vi "Autonomous State Machine.vi"   [LabVIEW 2014]
doc: "This VI is called when autonomous begins, and will automatically be terminated when autonomous ends. You can carry out timed or sensor driven robot movement independently without needing to return to the caller."
panel:
  # "Be sure to right-click and choose Data Operations>>Make Current Value default if you want to save the array values with the VI"
types:
  T1 = typedef "WPI_MotorControlDeviceRef.ctl" = cluster{"DeviceStatus":errorcluster, "Type":T2, "PWM":cluster{"Controller":T3, "PWM Channel":T4, "DeadBand":T5}, "CAN":cluster{"Device Number":u8, "Control Mode":T6, "Semaphore":T7, "Max Vout":dbl, "TalonSRX Control Mode":T8}, "Invert":bool, "TransformRef":T9, "InvTransformRef":T9}
  T2 = typedef "WPI_MotorControlType.ctl" = enum16{"PWM", "CAN", "CANTalonSRX"}
  T3 = typedef "FPGA_TypedefDigitalModule.ctl" = enum16{"Controller 1"}
  T4 = typedef "FPGA_DIOPWMChannel.ctl" = enum8{"PWM 0", "PWM 1", "PWM 2", "PWM 3", "PWM 4", "PWM 5", "PWM 6", "PWM 7", "PWM 8", "PWM 9", "PWM MXP 0", "PWM MXP 1", "PWM MXP 2", "PWM MXP 3", "PWM MXP 4", "PWM MXP 5", "PWM MXP 6", "PWM MXP 7", "PWM MXP 8", "PWM MXP 9", "Invalid"}
  T5 = typedef "WPI_PWMDeadband.ctl" = cluster{"Name":string, "maxPositivePwm":i32, "minPositivePwm":i32, "centerPwm":i32, "maxNegativePwm":i32, "minNegativePwm":i32, "angularRange":u16}
  T6 = typedef "WPI_CANJaguar_ControlMode.ctl" = enum8{"Percent VBus", "Current", "Speed", "Position", "Voltage"}
  T7 = typedef "Semaphore RefNum" = refnum<k1>
  T8 = typedef "WPI_CANTalonSRX_APIControlMode.ctl" = enum8{"Percent VBus", "Speed", "Position", "Slave", "Unchanged / Invalid"}
  T9 = typedef "WPI_PWMTransform_ConPane.ctl" = refnum<vi>
  T10 = typedef "WPI_DigitalInputDevRef.ctl" = cluster{"DevStatus":errorcluster, "DIO Channel":T11, "Controller":T3}
  T11 = typedef "FPGA_DIOChannel.ctl" = enum8{"DIO 0", "DIO 1", "DIO 2", "DIO 3", "DIO 4", "DIO 5", "DIO 6", "DIO 7", "DIO 8", "DIO 9", "DIO MXP 0", "DIO MXP 1", "DIO MXP 2", "DIO MXP 3", "DIO MXP 4", "DIO MXP 5", "DIO MXP 6", "DIO MXP 7", "DIO MXP 8", "DIO MXP 9", "DIO MXP 10", "DIO MXP 11", "DIO MXP 12", "DIO MXP 13", "DIO MXP 14", "DIO MXP 15", "Invalid"}
  T12 = typedef "WPI_RobotDriveDevRef.ctl" = cluster{"DevStatus":errorcluster, "Motors[]":T1[], "Square Inputs":bool, "Max Output":dbl}
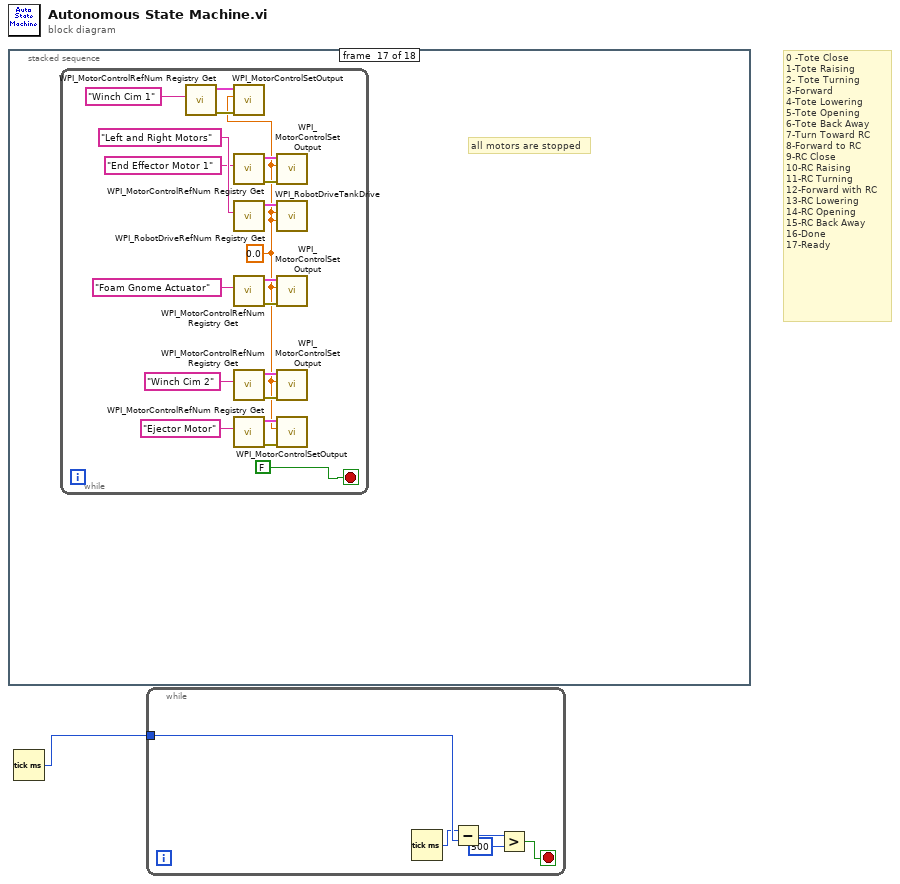
[diagram p0: block diagram]
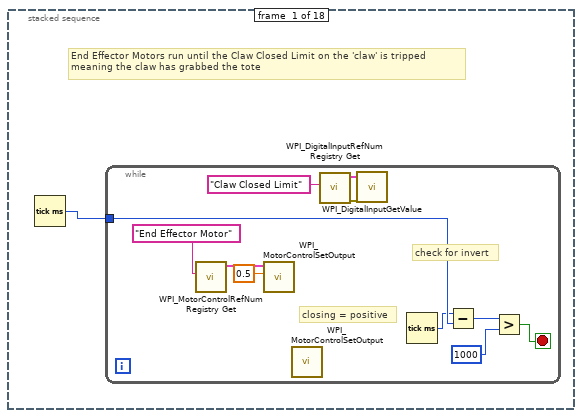
[diagram p2: hidden frame]
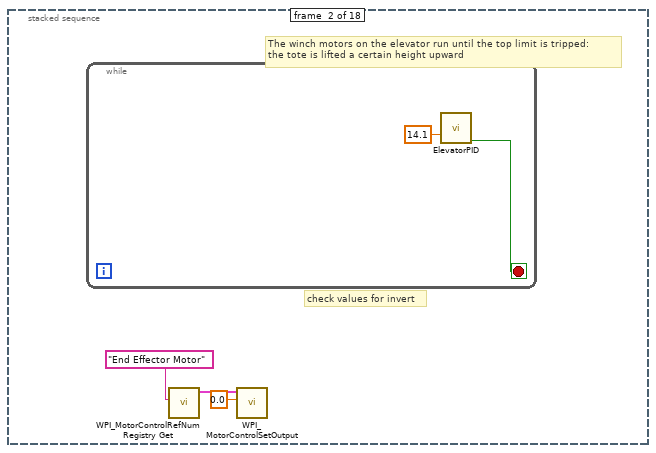
[diagram p3: hidden frame]
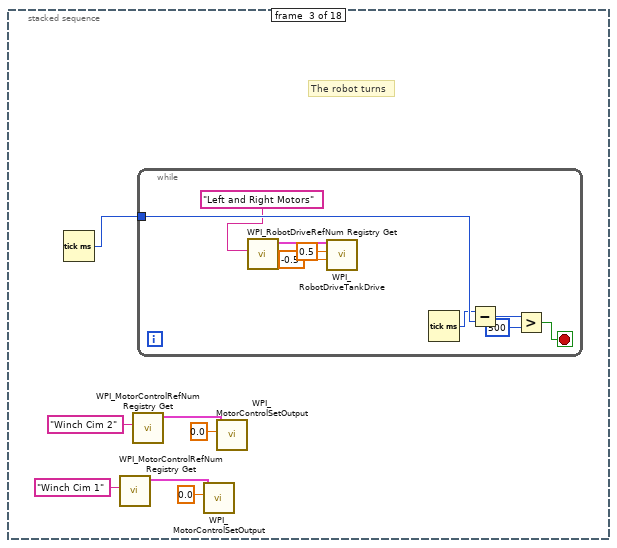
[diagram p4: hidden frame]
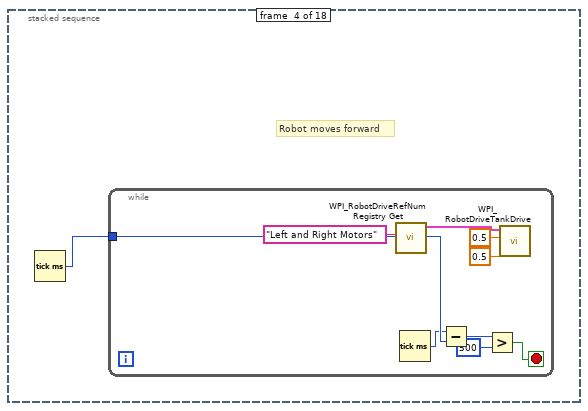
[diagram p5: hidden frame]
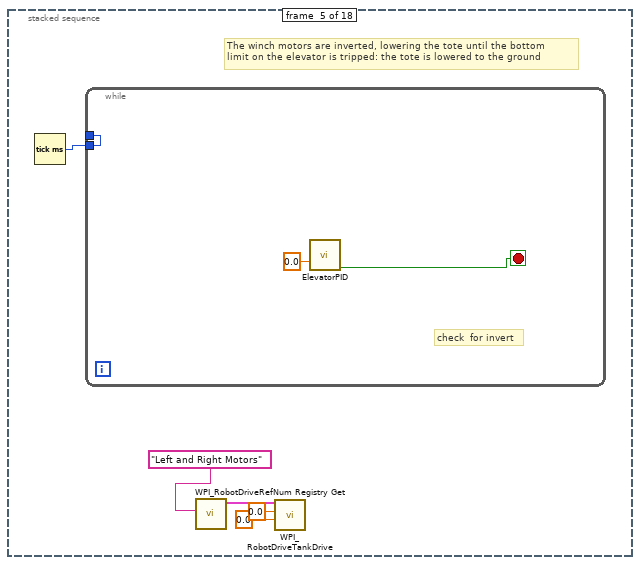
[diagram p6: hidden frame]
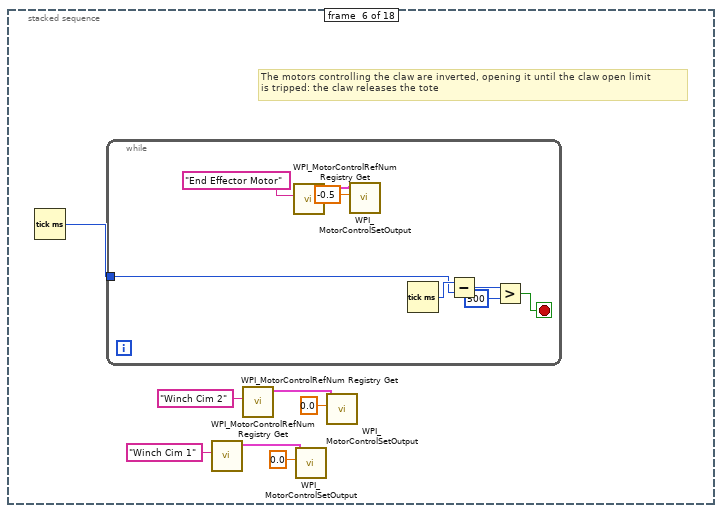
[diagram p7: hidden frame]
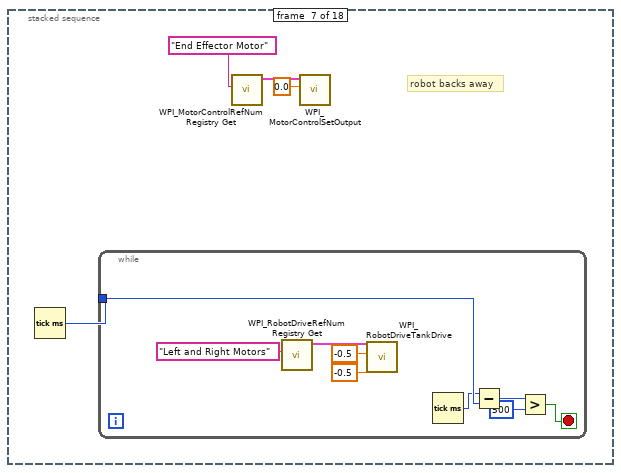
[diagram p8: hidden frame]
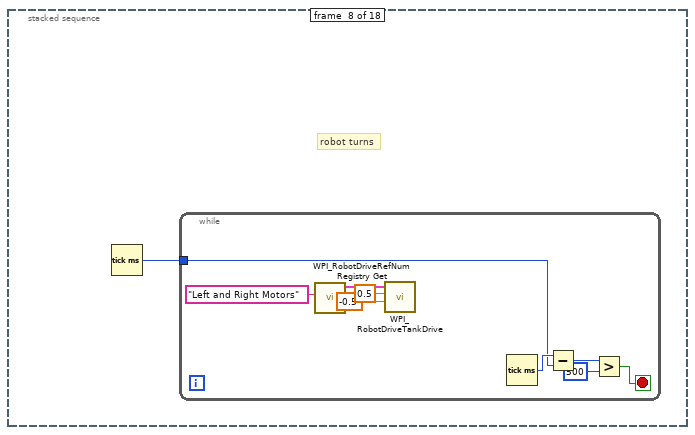
[diagram p9: hidden frame]
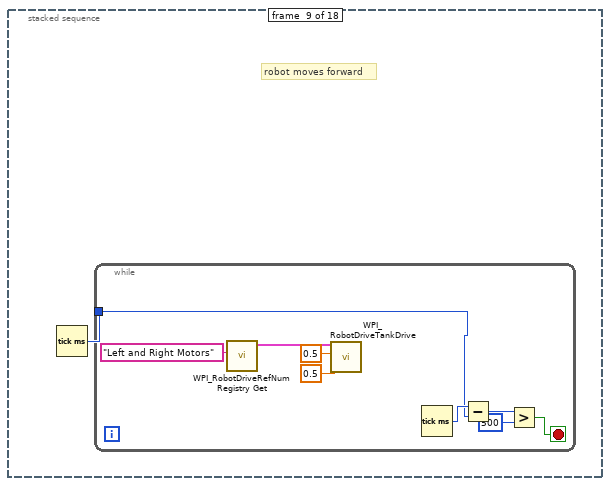
[diagram p10: hidden frame]
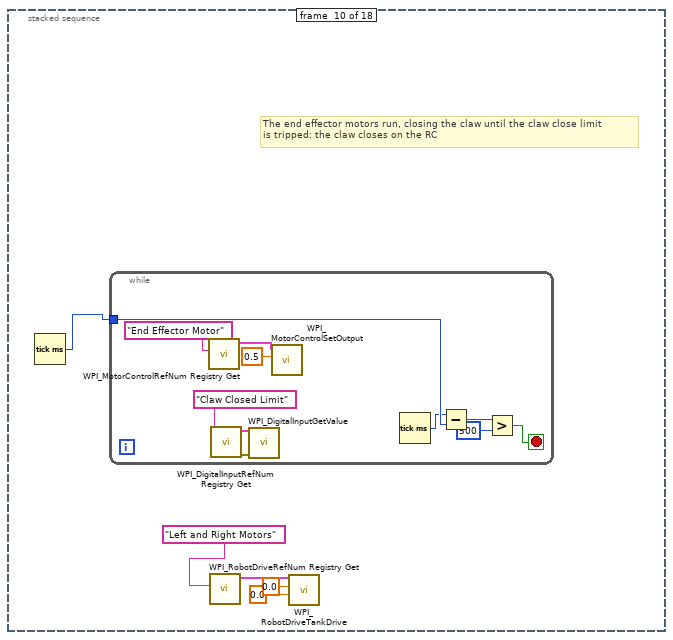
[diagram p11: hidden frame]
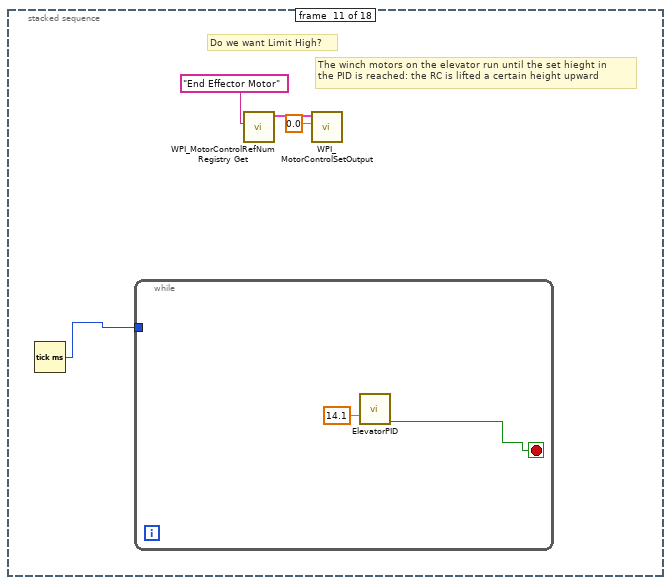
[diagram p12: hidden frame]
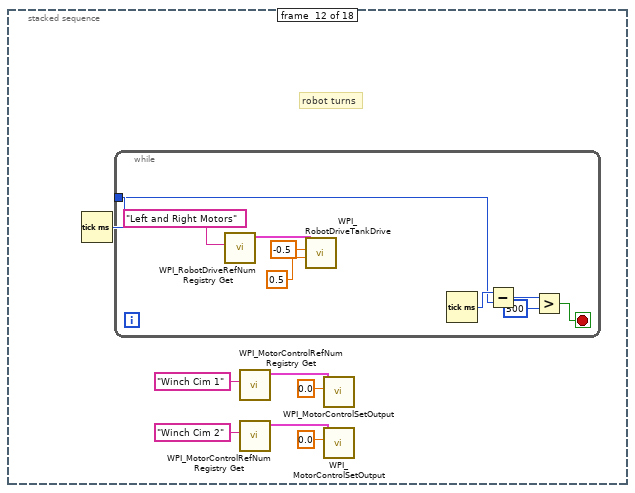
[diagram p13: hidden frame]
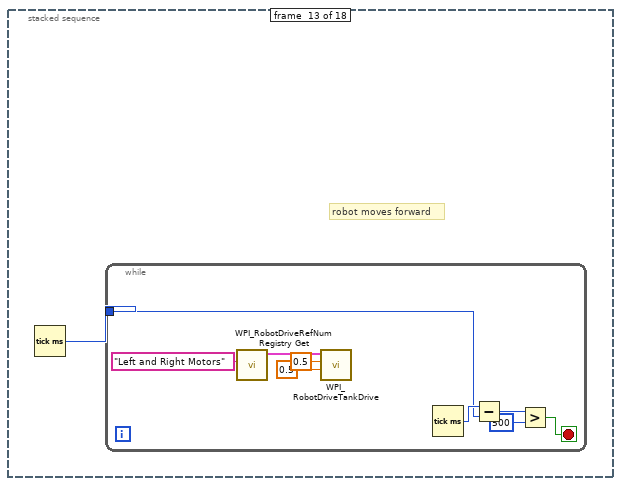
[diagram p14: hidden frame]
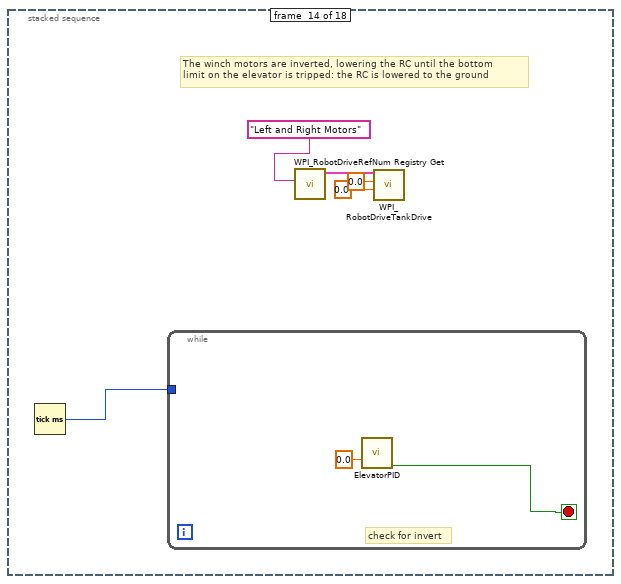
[diagram p15: hidden frame]
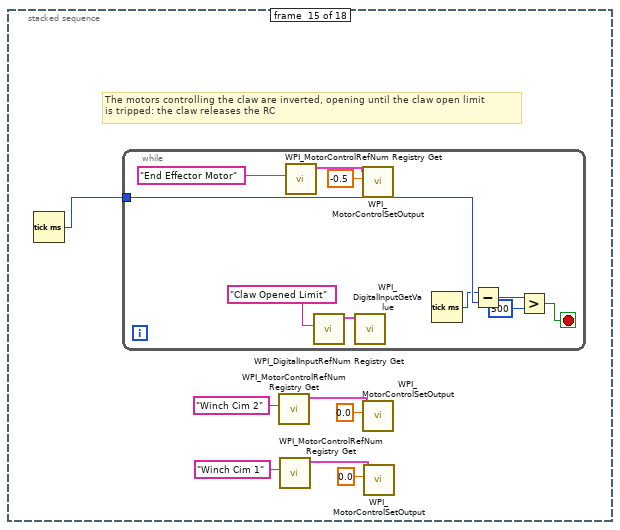
[diagram p16: hidden frame]
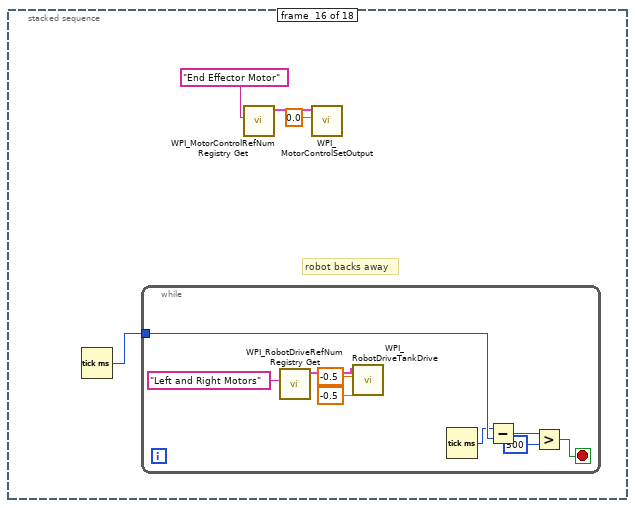
[diagram p17: hidden frame]
diagram:
  # "0 -Tote Close\n1-Tote Raising\n2- Tote Turning\n3-Forward\n4-Tote Lowering\n5-Tote Opening\n6-Tote Back Away\n7-Turn Toward RC\n8-Forward to RC\n9-RC Close\n10-RC Raising\n11-RC Turning\n12-Forward with RC\n13-RC Lowering\n14-RC Opening\n15-RC Back Away\n16-Done\n17-Ready"
  n1 = stacked-sequence {
    frame #0 {
      # "End Effector Motors run until the Claw Closed Limit on the 'claw' is tripped\nmeaning the claw has grabbed the tote"
      n2 = Tick Count (ms)() -> (millisecond timer value=w2:u32)
      n3 = while {
        tunnel: w2 -> [w10]
        stop <- w11 stop-if-true
        # "closing = positive"
        # "check for invert"
        n4 = call <vilib>:"WPI_MotorControlRefNum Registry Get.vi"("refnum name"="End Effector Motor") -> ("MotorControlDevRef"=w6:T1)  [unwired: 9 in, 1 out]
        n5 = call <vilib>:"WPI_MotorControlSetOutput.vi"("Output"=0.5, "MotorControlDevRef"=w6) -> ()  [unwired: 7 in, 3 out]
        n6 = call <vilib>:"WPI_MotorControlSetOutput.vi"() -> ()  [unwired: 9 in, 3 out]
        n7 = call <vilib>:"WPI_DigitalInputRefNum Registry Get.vi"("refnum name"="Claw Closed Limit") -> ("error out"=w4:errorcluster, "DigitalInputDevRef"=w3:T10)  [unwired: 9 in]
        n8 = call <vilib>:"WPI_DigitalInputGetValue.vi"("error in (no error)"=w4, "DigitalInputDevRef"=w3) -> ()  [unwired: 7 in, 3 out]
        n9 = Tick Count (ms)() -> (millisecond timer value=w9:u32)
        n10 = Subtract(x=w9, y=w10) -> (x-y=w13:u32)
        n11 = Greater?(x=w13, y=u32 1000) -> (0:w11:bool)
      }
    }
    frame #1 {
      # "The winch motors on the elevator run until the top limit is tripped: \nthe tote is lifted a certain height upward"
      # "check values for invert"
      n12 = while {
        stop <- w18 stop-if-true
        n13 = call "ElevatorPID.vi"("Elevator Setpoint"=14.1) -> ("At Setpoint"=w18:bool)  [unwired: 14 in]
      }
      n14 = call <vilib>:"WPI_MotorControlRefNum Registry Get.vi"("refnum name"="End Effector Motor") -> ("MotorControlDevRef"=w14:T1)  [unwired: 9 in, 1 out]
      n15 = call <vilib>:"WPI_MotorControlSetOutput.vi"("Output"=0.0, "MotorControlDevRef"=w14) -> ()  [unwired: 7 in, 3 out]
    }
    frame #2 {
      # "The robot turns"
      n16 = Tick Count (ms)() -> (millisecond timer value=w25:u32)
      n17 = call <vilib>:"WPI_MotorControlRefNum Registry Get.vi"("refnum name"="Winch Cim 1") -> ("MotorControlDevRef"=w20:T1)  [unwired: 9 in, 1 out]
      n18 = call <vilib>:"WPI_MotorControlRefNum Registry Get.vi"("refnum name"="Winch Cim 2") -> ("MotorControlDevRef"=w23:T1)  [unwired: 9 in, 1 out]
      n19 = while {
        tunnel: w25 -> [w31]
        stop <- w32 stop-if-true
        n20 = call <vilib>:"WPI_RobotDriveRefNum Registry Get.vi"("refnum name"="Left and Right Motors") -> ("RobotDriveDevRef"=w29:T12)  [unwired: 9 in, 1 out]
        n21 = call <vilib>:"WPI_RobotDriveTankDrive.vi"("Right axis value"=-0.5, "Left axis value"=0.5, "RobotDriveDevRef"=w29) -> ()  [unwired: 6 in, 3 out]
        n22 = Tick Count (ms)() -> (millisecond timer value=w30:u32)
        n23 = Subtract(x=w30, y=w31) -> (x-y=w34:u32)
        n24 = Greater?(x=w34, y=u32 500) -> (0:w32:bool)
      }
      n25 = call <vilib>:"WPI_MotorControlSetOutput.vi"("Output"=0.0, "MotorControlDevRef"=w20) -> ()  [unwired: 7 in, 3 out]
      n26 = call <vilib>:"WPI_MotorControlSetOutput.vi"("Output"=0.0, "MotorControlDevRef"=w23) -> ()  [unwired: 7 in, 3 out]
    }
    frame #3 {
      # "Robot moves forward"
      n27 = Tick Count (ms)() -> (millisecond timer value=w35:u32)
      n28 = while {
        tunnel: w35 -> [w41]
        stop <- w42 stop-if-true
        n29 = call <vilib>:"WPI_RobotDriveRefNum Registry Get.vi"("refnum name"="Left and Right Motors") -> ("RobotDriveDevRef"=w39:T12)  [unwired: 9 in, 1 out]
        n30 = Tick Count (ms)() -> (millisecond timer value=w40:u32)
        n31 = Subtract(x=w40, y=w41) -> (x-y=w44:u32)
        n32 = Greater?(x=w44, y=u32 500) -> (0:w42:bool)
        n33 = call <vilib>:"WPI_RobotDriveTankDrive.vi"("Right axis value"=0.5, "Left axis value"=0.5, "RobotDriveDevRef"=w39) -> ()  [unwired: 6 in, 3 out]
      }
    }
    frame #4 {
      # "The winch motors are inverted, lowering the tote until the bottom \nlimit on the elevator is tripped: the tote is lowered to the ground"
      n34 = Tick Count (ms)() -> (millisecond timer value=w49:u32)
      n35 = while {
        tunnel: [w52] -> _
        tunnel: w49 -> [w52]
        stop <- w50 stop-if-true
        # "check  for invert"
        n36 = call "ElevatorPID.vi"("Elevator Setpoint"=0.0) -> ("At Setpoint"=w50:bool)  [unwired: 14 in]
      }
      n37 = call <vilib>:"WPI_RobotDriveRefNum Registry Get.vi"("refnum name"="Left and Right Motors") -> ("RobotDriveDevRef"=w48:T12)  [unwired: 9 in, 1 out]
      n38 = call <vilib>:"WPI_RobotDriveTankDrive.vi"("Right axis value"=0.0, "Left axis value"=0.0, "RobotDriveDevRef"=w48) -> ()  [unwired: 6 in, 3 out]
    }
    frame #5 {
      # "The motors controlling the claw are inverted, opening it until the claw open limit\nis tripped: the claw releases the tote"
      n39 = Tick Count (ms)() -> (millisecond timer value=w59:u32)
      n40 = while {
        tunnel: w59 -> [w60]
        stop <- w65 stop-if-true
        n41 = call <vilib>:"WPI_MotorControlRefNum Registry Get.vi"("refnum name"="End Effector Motor") -> ("MotorControlDevRef"=w62:T1)  [unwired: 9 in, 1 out]
        n42 = call <vilib>:"WPI_MotorControlSetOutput.vi"("Output"=-0.5, "MotorControlDevRef"=w62) -> ()  [unwired: 7 in, 3 out]
        n43 = Tick Count (ms)() -> (millisecond timer value=w64:u32)
        n44 = Subtract(x=w64, y=w60) -> (x-y=w67:u32)
        n45 = Greater?(x=w67, y=u32 500) -> (0:w65:bool)
      }
      n46 = call <vilib>:"WPI_MotorControlRefNum Registry Get.vi"("refnum name"="Winch Cim 1") -> ("MotorControlDevRef"=w54:T1)  [unwired: 9 in, 1 out]
      n47 = call <vilib>:"WPI_MotorControlRefNum Registry Get.vi"("refnum name"="Winch Cim 2") -> ("MotorControlDevRef"=w57:T1)  [unwired: 9 in, 1 out]
      n48 = call <vilib>:"WPI_MotorControlSetOutput.vi"("Output"=0.0, "MotorControlDevRef"=w54) -> ()  [unwired: 7 in, 3 out]
      n49 = call <vilib>:"WPI_MotorControlSetOutput.vi"("Output"=0.0, "MotorControlDevRef"=w57) -> ()  [unwired: 7 in, 3 out]
    }
    frame #6 {
      # "robot backs away"
      n50 = Tick Count (ms)() -> (millisecond timer value=w71:u32)
      n51 = while {
        tunnel: w71 -> [w77]
        stop <- w78 stop-if-true
        n52 = call <vilib>:"WPI_RobotDriveRefNum Registry Get.vi"("refnum name"="Left and Right Motors") -> ("RobotDriveDevRef"=w75:T12)  [unwired: 9 in, 1 out]
        n53 = call <vilib>:"WPI_RobotDriveTankDrive.vi"("Right axis value"=-0.5, "Left axis value"=-0.5, "RobotDriveDevRef"=w75) -> ()  [unwired: 6 in, 3 out]
        n54 = Tick Count (ms)() -> (millisecond timer value=w76:u32)
        n55 = Subtract(x=w76, y=w77) -> (x-y=w80:u32)
        n56 = Greater?(x=w80, y=u32 500) -> (0:w78:bool)
      }
      n57 = call <vilib>:"WPI_MotorControlRefNum Registry Get.vi"("refnum name"="End Effector Motor") -> ("MotorControlDevRef"=w68:T1)  [unwired: 9 in, 1 out]
      n58 = call <vilib>:"WPI_MotorControlSetOutput.vi"("Output"=0.0, "MotorControlDevRef"=w68) -> ()  [unwired: 7 in, 3 out]
    }
    frame #7 {
      # "robot turns"
      n59 = Tick Count (ms)() -> (millisecond timer value=w81:u32)
      n60 = while {
        tunnel: w81 -> [w86]
        stop <- w88 stop-if-true
        n61 = call <vilib>:"WPI_RobotDriveRefNum Registry Get.vi"("refnum name"="Left and Right Motors") -> ("RobotDriveDevRef"=w85:T12)  [unwired: 9 in, 1 out]
        n62 = call <vilib>:"WPI_RobotDriveTankDrive.vi"("Right axis value"=-0.5, "Left axis value"=0.5, "RobotDriveDevRef"=w85) -> ()  [unwired: 6 in, 3 out]
        n63 = Tick Count (ms)() -> (millisecond timer value=w87:u32)
        n64 = Subtract(x=w87, y=w86) -> (x-y=w90:u32)
        n65 = Greater?(x=w90, y=u32 500) -> (0:w88:bool)
      }
    }
    frame #8 {
      # "robot moves forward"
      n66 = Tick Count (ms)() -> (millisecond timer value=w91:u32)
      n67 = while {
        tunnel: w91 -> [w96]
        stop <- w98 stop-if-true
        n68 = call <vilib>:"WPI_RobotDriveRefNum Registry Get.vi"("refnum name"="Left and Right Motors") -> ("RobotDriveDevRef"=w95:T12)  [unwired: 9 in, 1 out]
        n69 = call <vilib>:"WPI_RobotDriveTankDrive.vi"("Right axis value"=0.5, "Left axis value"=0.5, "RobotDriveDevRef"=w95) -> ()  [unwired: 6 in, 3 out]
        n70 = Tick Count (ms)() -> (millisecond timer value=w97:u32)
        n71 = Subtract(x=w97, y=w96) -> (x-y=w100:u32)
        n72 = Greater?(x=w100, y=u32 500) -> (0:w98:bool)
      }
    }
    frame #9 {
      # "The end effector motors run, closing the claw until the claw close limit \nis tripped: the claw closes on the RC"
      n73 = Tick Count (ms)() -> (millisecond timer value=w105:u32)
      n74 = while {
        tunnel: w105 -> [w113]
        stop <- w114 stop-if-true
        n75 = call <vilib>:"WPI_MotorControlRefNum Registry Get.vi"("refnum name"="End Effector Motor") -> ("MotorControlDevRef"=w109:T1)  [unwired: 9 in, 1 out]
        n76 = call <vilib>:"WPI_DigitalInputRefNum Registry Get.vi"("refnum name"="Claw Closed Limit") -> ("error out"=w107:errorcluster, "DigitalInputDevRef"=w108:T10)  [unwired: 9 in]
        n77 = call <vilib>:"WPI_DigitalInputGetValue.vi"("error in (no error)"=w107, "DigitalInputDevRef"=w108) -> ()  [unwired: 7 in, 3 out]
        n78 = call <vilib>:"WPI_MotorControlSetOutput.vi"("Output"=0.5, "MotorControlDevRef"=w109) -> ()  [unwired: 7 in, 3 out]
        n79 = Tick Count (ms)() -> (millisecond timer value=w112:u32)
        n80 = Subtract(x=w112, y=w113) -> (x-y=w116:u32)
        n81 = Greater?(x=w116, y=u32 500) -> (0:w114:bool)
      }
      n82 = call <vilib>:"WPI_RobotDriveRefNum Registry Get.vi"("refnum name"="Left and Right Motors") -> ("RobotDriveDevRef"=w104:T12)  [unwired: 9 in, 1 out]
      n83 = call <vilib>:"WPI_RobotDriveTankDrive.vi"("Right axis value"=0.0, "Left axis value"=0.0, "RobotDriveDevRef"=w104) -> ()  [unwired: 6 in, 3 out]
    }
    frame #10 {
      # "The winch motors on the elevator run until the set hieght in \nthe PID is reached: the RC is lifted a certain height upward"
      # "Do we want Limit High?"
      n84 = Tick Count (ms)() -> (millisecond timer value=w120:u32)
      n85 = while {
        tunnel: w120 -> [_]
        stop <- w121 stop-if-true
        n86 = call "ElevatorPID.vi"("Elevator Setpoint"=14.1) -> ("At Setpoint"=w121:bool)  [unwired: 14 in]
      }
      n87 = call <vilib>:"WPI_MotorControlRefNum Registry Get.vi"("refnum name"="End Effector Motor") -> ("MotorControlDevRef"=w119:T1)  [unwired: 9 in, 1 out]
      n88 = call <vilib>:"WPI_MotorControlSetOutput.vi"("Output"=0.0, "MotorControlDevRef"=w119) -> ()  [unwired: 7 in, 3 out]
    }
    frame #11 {
      # "robot turns"
      n89 = Tick Count (ms)() -> (millisecond timer value=w129:u32)
      n90 = while {
        tunnel: w129 -> [w134]
        stop <- w136 stop-if-true
        n91 = call <vilib>:"WPI_RobotDriveRefNum Registry Get.vi"("refnum name"="Left and Right Motors") -> ("RobotDriveDevRef"=w133:T12)  [unwired: 9 in, 1 out]
        n92 = call <vilib>:"WPI_RobotDriveTankDrive.vi"("Right axis value"=0.5, "Left axis value"=-0.5, "RobotDriveDevRef"=w133) -> ()  [unwired: 6 in, 3 out]
        n93 = Tick Count (ms)() -> (millisecond timer value=w135:u32)
        n94 = Subtract(x=w135, y=w134) -> (x-y=w138:u32)
        n95 = Greater?(x=w138, y=u32 500) -> (0:w136:bool)
      }
      n96 = call <vilib>:"WPI_MotorControlRefNum Registry Get.vi"("refnum name"="Winch Cim 1") -> ("MotorControlDevRef"=w127:T1)  [unwired: 9 in, 1 out]
      n97 = call <vilib>:"WPI_MotorControlRefNum Registry Get.vi"("refnum name"="Winch Cim 2") -> ("MotorControlDevRef"=w124:T1)  [unwired: 9 in, 1 out]
      n98 = call <vilib>:"WPI_MotorControlSetOutput.vi"("Output"=0.0, "MotorControlDevRef"=w127) -> ()  [unwired: 7 in, 3 out]
      n99 = call <vilib>:"WPI_MotorControlSetOutput.vi"("Output"=0.0, "MotorControlDevRef"=w124) -> ()  [unwired: 7 in, 3 out]
    }
    frame #12 {
      # "robot moves forward"
      n100 = Tick Count (ms)() -> (millisecond timer value=w139:u32)
      n101 = while {
        tunnel: w139 -> [w144]
        stop <- w146 stop-if-true
        n102 = call <vilib>:"WPI_RobotDriveRefNum Registry Get.vi"("refnum name"="Left and Right Motors") -> ("RobotDriveDevRef"=w143:T12)  [unwired: 9 in, 1 out]
        n103 = call <vilib>:"WPI_RobotDriveTankDrive.vi"("Right axis value"=0.5, "Left axis value"=0.5, "RobotDriveDevRef"=w143) -> ()  [unwired: 6 in, 3 out]
        n104 = Tick Count (ms)() -> (millisecond timer value=w145:u32)
        n105 = Subtract(x=w145, y=w144) -> (x-y=w148:u32)
        n106 = Greater?(x=w148, y=u32 500) -> (0:w146:bool)
      }
    }
    frame #13 {
      # "The winch motors are inverted, lowering the RC until the bottom \nlimit on the elevator is tripped: the RC is lowered to the ground"
      n107 = Tick Count (ms)() -> (millisecond timer value=w153:u32)
      n108 = while {
        tunnel: w153 -> [_]
        stop <- w154 stop-if-true
        # "check for invert"
        n109 = call "ElevatorPID.vi"("Elevator Setpoint"=0.0) -> ("At Setpoint"=w154:bool)  [unwired: 14 in]
      }
      n110 = call <vilib>:"WPI_RobotDriveRefNum Registry Get.vi"("refnum name"="Left and Right Motors") -> ("RobotDriveDevRef"=w152:T12)  [unwired: 9 in, 1 out]
      n111 = call <vilib>:"WPI_RobotDriveTankDrive.vi"("Right axis value"=0.0, "Left axis value"=0.0, "RobotDriveDevRef"=w152) -> ()  [unwired: 6 in, 3 out]
    }
    frame #14 {
      # "The motors controlling the claw are inverted, opening until the claw open limit\nis tripped: the claw releases the RC"
      n112 = Tick Count (ms)() -> (millisecond timer value=w162:u32)
      n113 = while {
        tunnel: w162 -> [w169]
        stop <- w170 stop-if-true
        n114 = call <vilib>:"WPI_MotorControlRefNum Registry Get.vi"("refnum name"="End Effector Motor") -> ("MotorControlDevRef"=w163:T1)  [unwired: 9 in, 1 out]
        n115 = call <vilib>:"WPI_DigitalInputRefNum Registry Get.vi"("refnum name"="Claw Opened Limit") -> ("DigitalInputDevRef"=w166:T10)  [unwired: 9 in, 1 out]
        n116 = call <vilib>:"WPI_DigitalInputGetValue.vi"("DigitalInputDevRef"=w166) -> ()  [unwired: 8 in, 3 out]
        n117 = call <vilib>:"WPI_MotorControlSetOutput.vi"("Output"=-0.5, "MotorControlDevRef"=w163) -> ()  [unwired: 7 in, 3 out]
        n118 = Tick Count (ms)() -> (millisecond timer value=w168:u32)
        n119 = Subtract(x=w168, y=w169) -> (x-y=w172:u32)
        n120 = Greater?(x=w172, y=u32 500) -> (0:w170:bool)
      }
      n121 = call <vilib>:"WPI_MotorControlRefNum Registry Get.vi"("refnum name"="Winch Cim 2") -> ("MotorControlDevRef"=w160:T1)  [unwired: 9 in, 1 out]
      n122 = call <vilib>:"WPI_MotorControlRefNum Registry Get.vi"("refnum name"="Winch Cim 1") -> ("MotorControlDevRef"=w157:T1)  [unwired: 9 in, 1 out]
      n123 = call <vilib>:"WPI_MotorControlSetOutput.vi"("Output"=0.0, "MotorControlDevRef"=w160) -> ()  [unwired: 7 in, 3 out]
      n124 = call <vilib>:"WPI_MotorControlSetOutput.vi"("Output"=0.0, "MotorControlDevRef"=w157) -> ()  [unwired: 7 in, 3 out]
    }
    frame #15 {
      # "robot backs away"
      n125 = Tick Count (ms)() -> (millisecond timer value=w176:u32)
      n126 = while {
        tunnel: w176 -> [w182]
        stop <- w183 stop-if-true
        n127 = call <vilib>:"WPI_RobotDriveRefNum Registry Get.vi"("refnum name"="Left and Right Motors") -> ("RobotDriveDevRef"=w180:T12)  [unwired: 9 in, 1 out]
        n128 = call <vilib>:"WPI_RobotDriveTankDrive.vi"("Right axis value"=-0.5, "Left axis value"=-0.5, "RobotDriveDevRef"=w180) -> ()  [unwired: 6 in, 3 out]
        n129 = Tick Count (ms)() -> (millisecond timer value=w181:u32)
        n130 = Subtract(x=w181, y=w182) -> (x-y=w185:u32)
        n131 = Greater?(x=w185, y=u32 500) -> (0:w183:bool)
      }
      n132 = call <vilib>:"WPI_MotorControlRefNum Registry Get.vi"("refnum name"="End Effector Motor") -> ("MotorControlDevRef"=w173:T1)  [unwired: 9 in, 1 out]
      n133 = call <vilib>:"WPI_MotorControlSetOutput.vi"("Output"=0.0, "MotorControlDevRef"=w173) -> ()  [unwired: 7 in, 3 out]
    }
    frame #16 {
      # "all motors are stopped"
      n134 = while {
        stop <- FALSE stop-if-true
        w186 = 0.0
        n135 = call <vilib>:"WPI_MotorControlRefNum Registry Get.vi"("refnum name"="Winch Cim 1") -> ("error out"=w195:errorcluster, "MotorControlDevRef"=w194:T1)  [unwired: 9 in]
        n136 = call <vilib>:"WPI_MotorControlSetOutput.vi"("error in (no error)"=w195, "Output"=w186, "MotorControlDevRef"=w194) -> ()  [unwired: 6 in, 3 out]
        n137 = call <vilib>:"WPI_MotorControlRefNum Registry Get.vi"("refnum name"="End Effector Motor 1") -> ("error out"=w201:errorcluster, "MotorControlDevRef"=w200:T1)  [unwired: 9 in]
        n138 = call <vilib>:"WPI_RobotDriveRefNum Registry Get.vi"("refnum name"="Left and Right Motors") -> ("RobotDriveDevRef"=w203:T12)  [unwired: 9 in, 1 out]
        n139 = call <vilib>:"WPI_MotorControlRefNum Registry Get.vi"("refnum name"="Foam Gnome Actuator") -> ("error out"=w199:errorcluster, "MotorControlDevRef"=w198:T1)  [unwired: 9 in]
        n140 = call <vilib>:"WPI_MotorControlRefNum Registry Get.vi"("refnum name"="Winch Cim 2") -> ("error out"=w197:errorcluster, "MotorControlDevRef"=w196:T1)  [unwired: 9 in]
        n141 = call <vilib>:"WPI_MotorControlRefNum Registry Get.vi"("refnum name"="Ejector Motor") -> ("error out"=w191:errorcluster, "MotorControlDevRef"=w190:T1)  [unwired: 9 in]
        n142 = call <vilib>:"WPI_MotorControlSetOutput.vi"("error in (no error)"=w201, "Output"=w186, "MotorControlDevRef"=w200) -> ()  [unwired: 6 in, 3 out]
        n143 = call <vilib>:"WPI_RobotDriveTankDrive.vi"("Right axis value"=w186, "Left axis value"=w186, "RobotDriveDevRef"=w203) -> ()  [unwired: 6 in, 3 out]
        n144 = call <vilib>:"WPI_MotorControlSetOutput.vi"("error in (no error)"=w199, "Output"=w186, "MotorControlDevRef"=w198) -> ()  [unwired: 6 in, 3 out]
        n145 = call <vilib>:"WPI_MotorControlSetOutput.vi"("error in (no error)"=w197, "Output"=w186, "MotorControlDevRef"=w196) -> ()  [unwired: 6 in, 3 out]
        n146 = call <vilib>:"WPI_MotorControlSetOutput.vi"("error in (no error)"=w191, "Output"=w186, "MotorControlDevRef"=w190) -> ()  [unwired: 6 in, 3 out]
      }
    }
    frame #17 {
      # "absolutely nothing happens here"
    }
  }
  n147 = Tick Count (ms)() -> (millisecond timer value=w1:u32)
  n148 = while {
    tunnel: w1 -> [w206]
    stop <- w207 stop-if-true
    n149 = Tick Count (ms)() -> (millisecond timer value=w205:u32)
    n150 = Subtract(x=w205, y=w206) -> (x-y=w209:u32)
    n151 = Greater?(x=w209, y=u32 500) -> (0:w207:bool)
  }
